vi "Process AIs.vi"(10 "AI Ref In":T1) -> (0 "GRF R":dbl, 1 "GRF L":dbl, 2 "Motor Velocity":dbl, 3 "Actual Motor Current":dbl, 4 "error out":errorcluster, 5 "Vicon Trigger Signal":dbl)   [LabVIEW 2018]
uses:
  <vilib>/myRIO/Instrument Drivers/Onboard IO/AI/typedefs/AI Reference.ctl
  <vilib>/myRIO/Common/Instrument Driver Framework/Utilities/typedefs/myRIO Generic Hardware Reference.ctl
  <vilib>/myRIO/Common/Instrument Driver Framework/Utilities/typedefs/Hardware Version Enum.ctl
  <vilib>/myRIO/Common/Instrument Driver Framework/Utilities/typedefs/myRIO v1.0 Reference.ctl
  <vilib>/myRIO/Common/Instrument Driver Framework/Utilities/typedefs/Generic FPGA Reference.ctl
  <vilib>/myRIO/Common/Instrument Driver Framework/myRIO v1.0/AI/typedefs/AI Channels List.ctl
  <vilib>/myRIO/Common/Instrument Driver Framework/myRIO v1.0/AI/typedefs/AI Channels Enum.ctl
  <vilib>/myRIO/Common/Instrument Driver Framework/Utilities/typedefs/Analog Scaling Constants List.ctl
  <vilib>/myRIO/Common/Instrument Driver Framework/Utilities/typedefs/Analog Scaling Constants.ctl
  <vilib>/Utility/error.llb/Error Cluster From Error Code.vi
  <vilib>/myRIO/Common/Instrument Driver Framework/myRIO v1.0/AI/vis/myRIO v1.0 Read AI.vi
  <vilib>/myRIO/Instrument Drivers/Onboard IO/AI/AI.lvlib
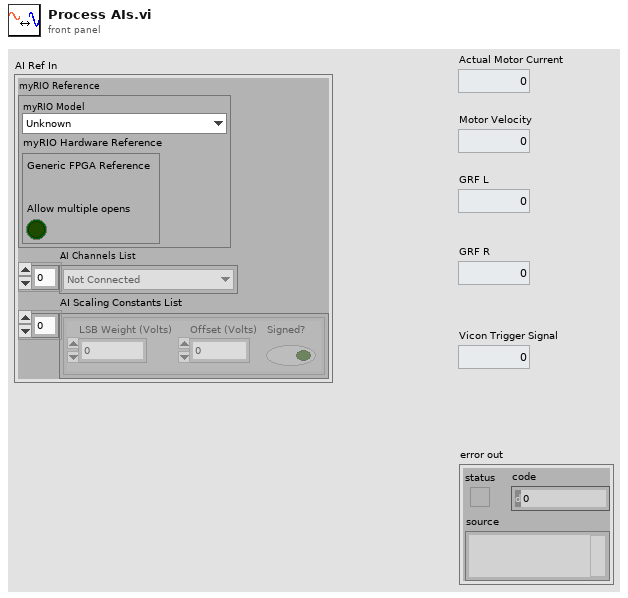
[diagram p1: front panel]
types:
  T1 = typedef "AI.lvlib/AI Reference.ctl" = cluster{"myRIO Reference":T2, "AI Channels List":T6, "AI Scaling Constants List":T8}
  T2 = typedef "myRIO Generic Hardware Reference.ctl" = cluster{"myRIO Model":T3, "myRIO Hardware Reference":T4}
  T3 = typedef "Hardware Version Enum.ctl" = enum16{"Unknown", "myRIO-1900", "myRIO-1950", "roboRIO", "NI ELVIS RIO CM", "ELVIS III"}
  T4 = typedef "myRIO v1.0 Reference.ctl" = cluster{"Generic FPGA Reference":T5, "Allow multiple opens":bool}
  T5 = typedef "Generic FPGA Reference.ctl" = refnum<k20>
  T6 = typedef "AI Channels List.ctl" = T7[]
  T7 = typedef "AI Channels Enum.ctl" = enum16{"Not Connected", "AudioIn/Left", "AudioIn/Right", "C/AI0", "C/AI1", "A/AI0", "A/AI1", "A/AI2", "A/AI3", "A/AI4", "A/AI5", "A/AI6", "A/AI7", "B/AI0", "B/AI1", "B/AI2", "B/AI3", "B/AI4", "B/AI5", "B/AI6", "B/AI7", "AI/AI0", "AI/AI1", "AI/AI2", "AI/AI3", "A/AI0 (DIFF)", "A/AI1 (DIFF)", "A/AI2 (DIFF)", "A/AI3 (DIFF)", "B/AI0 (DIFF)", "B/AI1 (DIFF)", "B/AI2 (DIFF)", "B/AI3 (DIFF)"}
  T8 = typedef "Analog Scaling Constants List.ctl" = T9[]
  T9 = typedef "Analog Scaling Constants.ctl" = cluster{"LSB Weight (Volts)":dbl, "Offset (Volts)":dbl, "Signed?":bool}
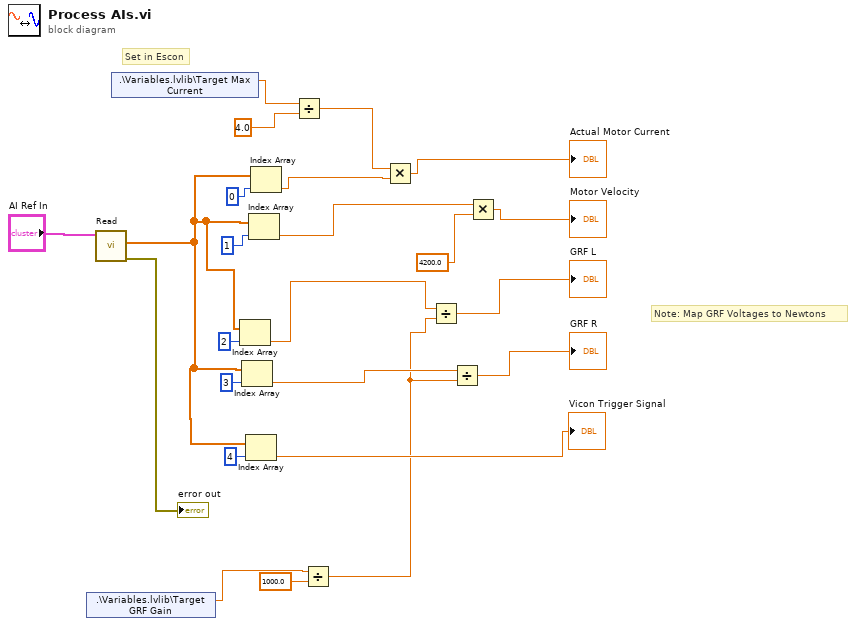
[diagram p0: block diagram]
diagram:
  # "Set in Escon"
  # "Note: Map GRF Voltages to Newtons"
  n1 = shared-variable ".\\Variables.lvlib\\Target GRF Gain"() -> (w3:dbl)  [unwired: 1 in, 1 out]
  n2 = call <vilib>:"Read.vi"("AI Ref In"="AI Ref In") -> ("error out"=→"error out":errorcluster, "Values"=w9:dbl[])  [unwired: 8 in, 1 out]
  n3 = shared-variable ".\\Variables.lvlib\\Target Max Current"() -> (w12:dbl)  [unwired: 1 in, 1 out]
  n4 = Index Array(array=w9, index=2) -> (element=w7:dbl)
  n5 = Index Array(array=w9, index=3) -> (element=w5:dbl)
  n6 = Index Array(array=w9, index=4) -> (element=→"Vicon Trigger Signal":dbl)
  n7 = Index Array(array=w9, index=1) -> (element=w17:dbl)
  n8 = Index Array(array=w9, index=0) -> (element=w19:dbl)
  n9 = Divide(x=w12, y=4.0) -> (x/y=w13:dbl)
  n10 = Divide(x=w3, y=1000.0) -> (x/y=w1:dbl)
  n11 = Multiply(x=w13, y=w19) -> (x*y=→"Actual Motor Current":dbl)
  n12 = Divide(x=w7, y=w1) -> (x/y=→"GRF L":dbl)
  n13 = Divide(x=w5, y=w1) -> (x/y=→"GRF R":dbl)
  n14 = Multiply(x=w17, y=4200.0) -> (x*y=→"Motor Velocity":dbl)
